vi "set_PulseDelay.vi"() -> ()   [LabVIEW 2014]
panel:
  in  "Address (0x50)":u16=80 max=1023 format="%.0x"
  in  "Aardvark Handle":i32 min=0
  out "error out":errorcluster
  in  "error in (no error)":errorcluster
  in  "Pulse Delay":dbl
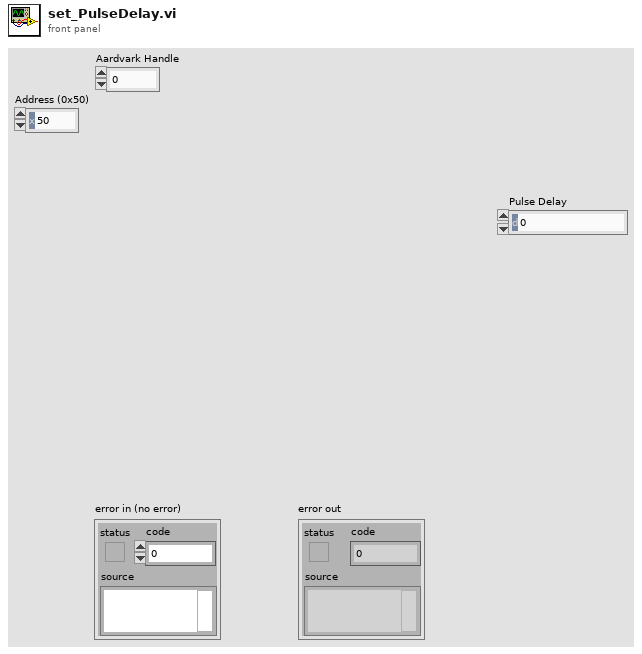
[diagram p1: front panel]
types:
  T1 = cluster{"unsigned byte array[0]":u8, "unsigned byte array[1]":u8, "unsigned byte array[2]":u8, "unsigned byte array[3]":u8, "unsigned byte array[4]":u8, "unsigned byte array[5]":u8, "unsigned byte array[6]":u8, "unsigned byte array[7]":u8, "unsigned byte array[8]":u8}
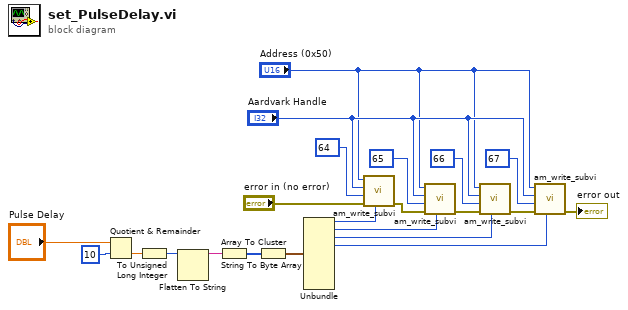
[diagram p0: block diagram]
diagram:
  n1 = Quotient & Remainder(x="Pulse Delay", y=10) -> (floor(x/y)=w19:dbl)  [unwired: 1 out]
  n2 = To Unsigned Long Integer(number=w19) -> (unsigned 32bit integer=w18:u32)
  n3 = Flatten To String(anything=w18) -> (data string=w20:string)  [unwired: 3 in, 2 out]
  n4 = String To Byte Array(string=w20) -> (unsigned byte array=w17:u8[])
  n5 = Array To Cluster(array=w17) -> (cluster=w16:T1)
  n6 = Unbundle(w16) -> ("unsigned byte array[0]"=w4:u8, "unsigned byte array[1]"=w3:u8, "unsigned byte array[2]"=w2:u8, "unsigned byte array[3]"=w1:u8)  [unwired: 5 out]
  n7 = call "am_write_subvi.vi"("Data to Write"=w4, "error in (no error)"="error in (no error)", "Memory ADD"=u16 64, "Aardvark Handle in"="Aardvark Handle", "Address (0x50) in"="Address (0x50)") -> ("error out"=w14:errorcluster)  [unwired: 5 in, 1 out]
  n8 = call "am_write_subvi.vi"("Data to Write"=w3, "error in (no error)"=w14, "Memory ADD"=u16 65, "Aardvark Handle in"="Aardvark Handle", "Address (0x50) in"="Address (0x50)") -> ("error out"=w11:errorcluster)  [unwired: 5 in, 1 out]
  n9 = call "am_write_subvi.vi"("Data to Write"=w2, "error in (no error)"=w11, "Memory ADD"=u16 66, "Aardvark Handle in"="Aardvark Handle", "Address (0x50) in"="Address (0x50)") -> ("error out"=w13:errorcluster)  [unwired: 5 in, 1 out]
  n10 = call "am_write_subvi.vi"("Data to Write"=w1, "error in (no error)"=w13, "Memory ADD"=u16 67, "Aardvark Handle in"="Aardvark Handle", "Address (0x50) in"="Address (0x50)") -> ("error out"=→"error out":errorcluster)  [unwired: 5 in, 1 out]
